vi "Main.vi"(11 "Module Admin":refnum<class "Delacor_lib_QMH_Module Admin.lvclass">) -> ()   [LabVIEW 2021, in "RT Interpreter Manager.lvlib"]
doc: "This template is based off of the Queued Message Handler design pattern and the Queued Message Handler project template that ships with LabVIEW.\n\nThe main difference is that the queue is private to this module and communication between modules is performed via Broadcast and Request events.\n\nRequest events are wrapped in public API methods and are handled in the Event Handling Loop (EHL) of this VI. Any module can register for Broadcast events sent by this module. The EHL generates messages based on user interface actions.\n\nThe Message Handling Loop (MHL) processes messages generated by the EHL, or by other messages. The messages are string values, so new messages can be added easily to the Message Cases case structure in the MHL. Each message cluster can also provide an optional value for Message Data, which is a variant that can be converted to whatever message-specific data is required.\n_____\nBased on DQMH Dev Tools: Project Template 7.1.2.1547."
uses:
  RT Interpreter Manager.lvlib
  <vilib>/Delacor/Delacor QMH/Libraries/Module Admin_class/Delacor_lib_QMH_Module Admin.lvclass
  Module Data--cluster.ctl
  Read Messages from Host HL--cluster.ctl
  Stop Argument--cluster.ctl
  <vilib>/Delacor/Delacor QMH/Libraries/Message Queue_class/Delacor_lib_QMH_Message Queue.lvclass/Delacor_lib_QMH_Message Queue.ctl
  <vilib>/Delacor/Delacor QMH/Libraries/Module Admin_class/Delacor_lib_QMH_Module Admin.lvclass/Delacor_lib_QMH_Module Admin.ctl
  New Host Connection Argument--cluster.ctl
  Send Message to Host Argument--cluster.ctl
  Libraries/UDP Comms/UDP Message--cluster.ctl
  Host/Host Interpreter/Host Initialization--cluster.ctl
  <vilib>/Utility/miscctls.llb/LVPointTypeDef.ctl
  0413ff4f-ab78-4adc-820c-bd9cd632877c.vi
  <vilib>/Delacor/Delacor QMH/Libraries/Message Queue_class/Delacor_lib_QMH_Enqueue Message (Single).vi
  <vilib>/Delacor/Delacor QMH/Libraries/Module Admin_class/Delacor_lib_QMH_Get External Launch.vi
  <vilib>/JDP Science/JSONtext/JSON text to Variant.vi
  <vilib>/JDP Science/JSONtext/LVClass Serializer/JSONtext LVClass Serializer.lvclass
  <vilib>/Delacor/Delacor QMH/Libraries/Message Queue_class/Delacor_lib_QMH_Message Queue.lvclass
  Libraries/Utilities/Utilities.lvlib
  RT Interpreter.lvlib
  Libraries/UDP Comms/UDP Comms.lvlib
  Libraries/Common RT/Common RT.lvlib
panel:
  out "error out":errorcluster
  out "Status":string
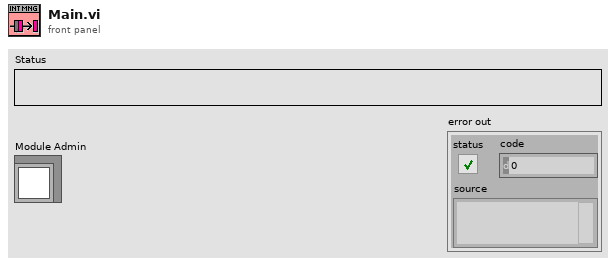
[diagram p1: front panel]
types:
  T1 = typedef "RT Interpreter Manager.lvlib/Request Events--cluster.ctl" = cluster{"Stop Module":refnum<user-event>, "Show Panel":refnum<user-event>, "Hide Panel":refnum<user-event>, "Get Module Execution Status":refnum<user-event>, "Show Diagram":refnum<user-event>, "Private.Get Config":refnum<user-event>, "Private.Open UDP":refnum<user-event>, "Private.Start Read Messages from Host HL":refnum<user-event>, "Private.New Host Connection":refnum<user-event>, "Private.Send Message to Host":refnum<user-event>, "Private.Delete Host Connection":refnum<user-event>}
  T2 = typedef "RT Interpreter Manager.lvlib/Read Messages from Host HL--cluster.ctl" = cluster{"Target UDP connection ID":refnum<k16>}
  T3 = typedef "RT Interpreter Manager.lvlib/Module Data--cluster.ctl" = cluster{"Status":string, "Target IP":string, "Target Listening Port":u16, "Polling Rate (ms)":i32, "UDP Connected?":bool, "Target UDP connection ID":refnum<k16>, "Host Connections IP:Port:Master/Slave":string[]}
  T4 = typedef "UDP Comms.lvlib/Host Initialization--cluster.ctl" = cluster{"Host IP":string, "Host Listening Port":u16, "MasterHost?":bool}
  T5 = enum32{"invalid lock state", "Not Locked", "Locked (No Password)", "Password-protected"}
  T6 = typedef "RT Interpreter Manager.lvlib/Stop Argument--cluster.ctl" = cluster{"Origin":string, "Exit via Stop Module Req?":bool, "Wait for Module to stop?":bool}
  T7 = typedef "RT Interpreter Manager.lvlib/New Host Connection Argument--cluster.ctl" = cluster{"Host Connection IP:Port:Master/Slave":string}
  T8 = typedef "RT Interpreter Manager.lvlib/Send Message to Host Argument--cluster.ctl" = cluster{"UDP Message":T9, "Remote IP":string, "Remote UDP Listening Port":u16}
  T9 = typedef "UDP Comms.lvlib/UDP Message--cluster.ctl" = cluster{"Command":string, "Data":variant}
  T10 = typedef "LVPointTypeDef.ctl" = cluster{"Horizontal":i16, "Vertical":i16}
  T11 = enum32{"Invalid", "Standard", "Closed", "Hidden", "Minimized", "Maximized"}
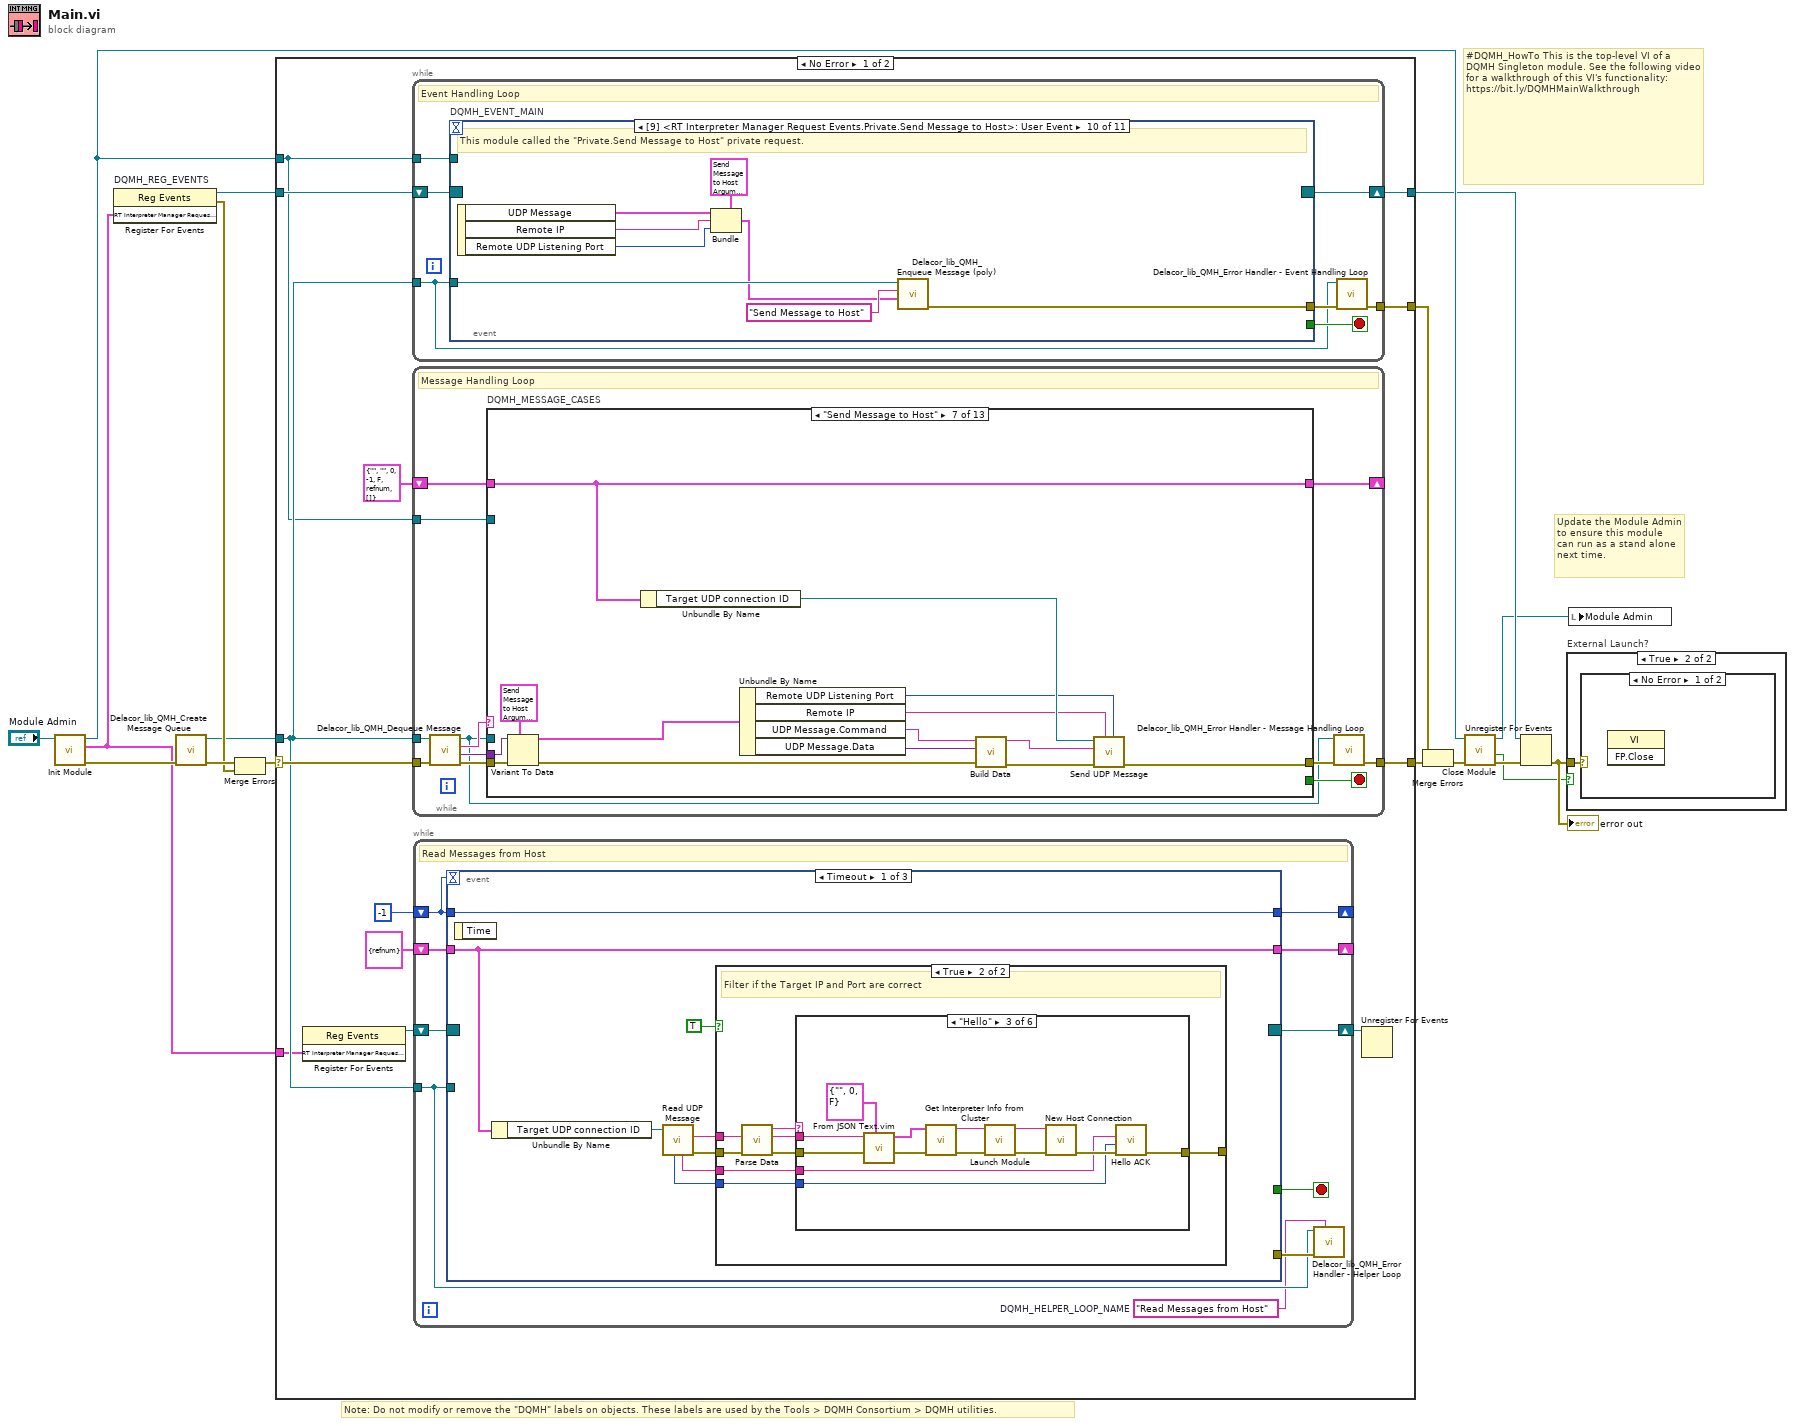
[diagram p0: block diagram]
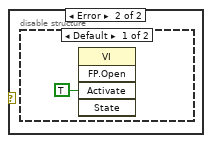
[diagram p3: hidden frame]
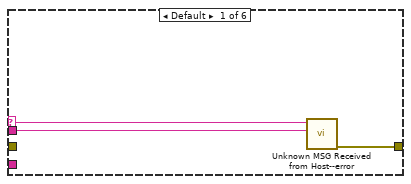
[diagram p6: hidden frame]
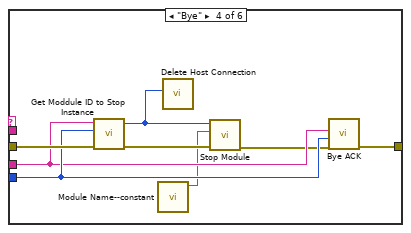
[diagram p8: hidden frame]
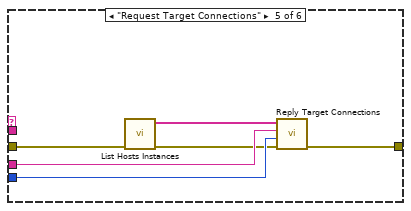
[diagram p9: hidden frame]
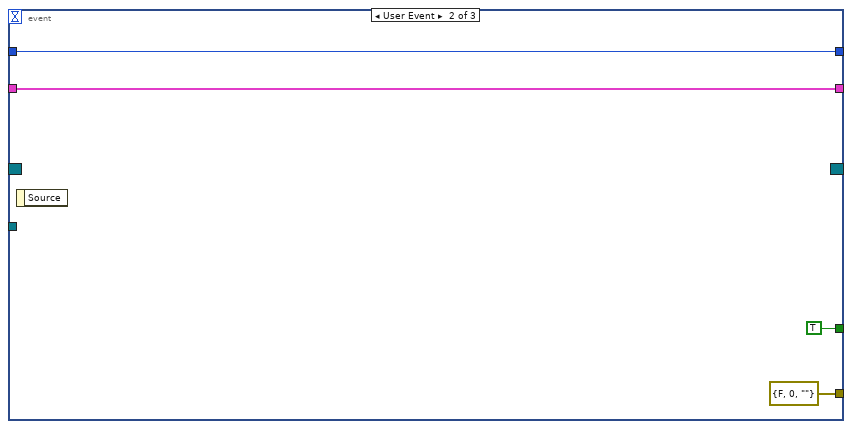
[diagram p11: hidden frame]
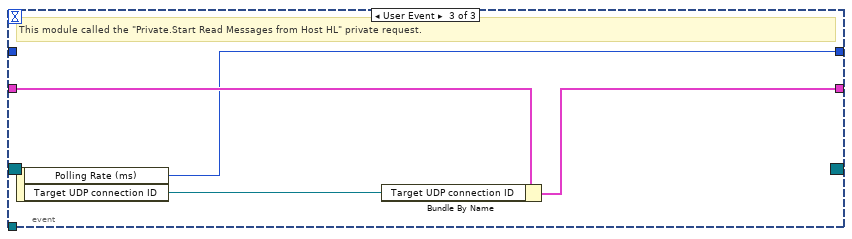
[diagram p12: hidden frame]
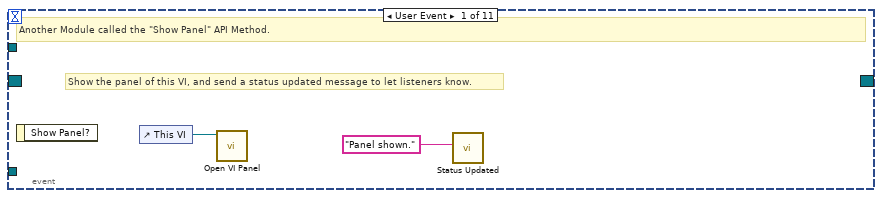
[diagram p13: hidden frame]
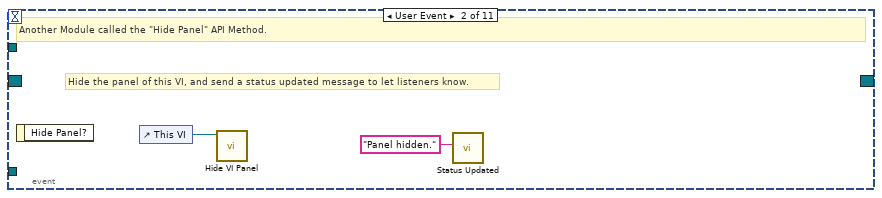
[diagram p14: hidden frame]
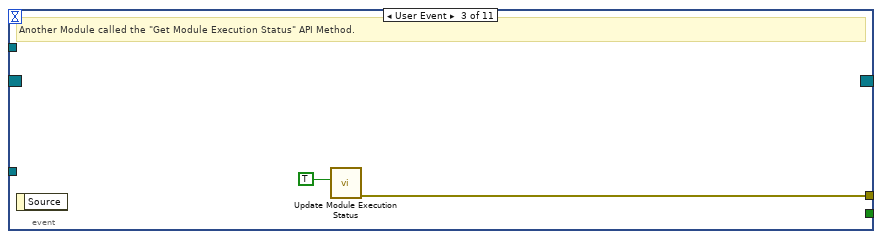
[diagram p15: hidden frame]
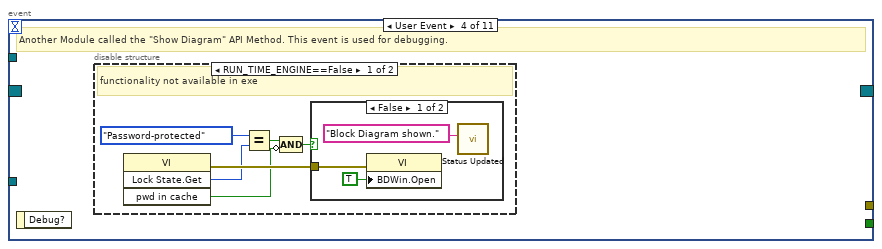
[diagram p16: hidden frame]
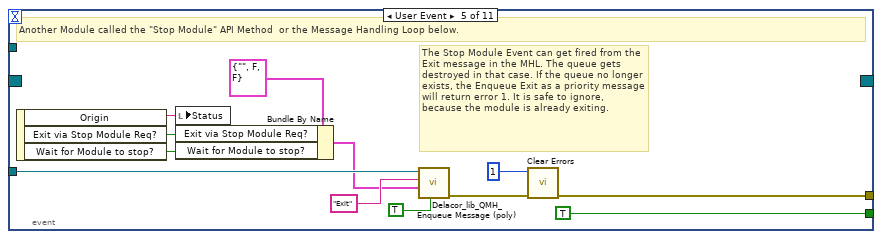
[diagram p19: hidden frame]
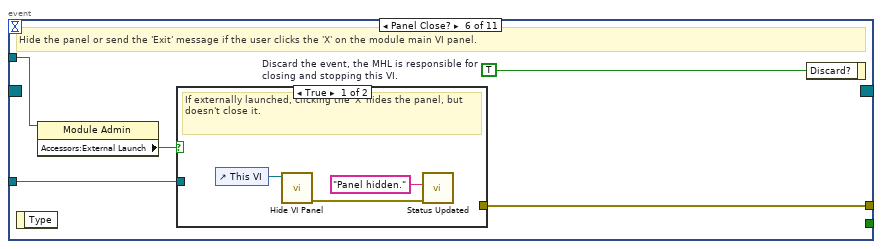
[diagram p20: hidden frame]
diagram:
  # "#DQMH_HowTo This is the top-level VI of a DQMH Singleton module. See the following video for a walkthrough of this VI's functionality: https://bit.ly/DQMHMainWalkthrough"
  # "Note: Do not modify or remove the \"DQMH\" labels on objects. These labels are used by the Tools > DQMH Consortium > DQMH utilities."
  # "Update the Module Admin to ensure this module can run as a stand alone next time."
  n1 = call "Init Module.vi"("Singleton Module Admin in"="Module Admin") -> ("error out"=w16:errorcluster, "RT Interpreter Manager Request Events"=w1:T1, "Singleton Module Admin out"=w8:refnum<class "Delacor_lib_QMH_Module Admin.lvclass">)  [unwired: 8 in]
  n2 = register-events "DQMH_REG_EVENTS"(w1) -> (reference out=w6:refnum<event-registration>, error out=w9:errorcluster)  [unwired: 2 in]
  n3 = call <vilib>:"Delacor_lib_QMH_Create Message Queue.vi"("error in"=w16) -> ("error out"=w11:errorcluster, "Message Queue"=w5:refnum<class "Delacor_lib_QMH_Message Queue.lvclass">)  [unwired: 9 in]
  n4 = Merge Errors(w11, w9) -> (w10:errorcluster)
  n5 = case shown="No Error" w10 {
    selector: w10 -> [w28 w316]
    tunnel: [w30 w315] -> w17
    tunnel: [w27 w314] -> w7
    tunnel: w6 -> [w25 w314]
    tunnel: w5 -> [w24 w309]
    tunnel: [w29 _] -> w14
    tunnel: w8 -> [w23 w310]
    tunnel: w1 -> [w22 _]
    frame No Error {
      n6 = register-events ("DQMH_HELPER_REGFOREVENTS")(w22) -> (reference out=w20:refnum<event-registration>)  [unwired: 2 in, 1 out]
      n7 = while {
        tunnel: w24 -> [w98]
        shift-right: [w101] -> w27
        shift-left: w25 -> [w102]
        tunnel: [w103] -> w29
        tunnel: w23 -> [w99]
        stop <- w100 stop-if-true
        # "Event Handling Loop"
        n8 = event "DQMH_EVENT_MAIN" shown="[9] <RT Interpreter Manager Request Events.Private.Send Message to Host>: User Event" {
          selector: w102 -> [_ _ _ _ _ _ _ _ _ _ _]
          dyn-events: [_ _ _ _ _ _ _ _ _ _ _] -> w101
          timeout: _ -> [_ _ _ _ _ _ _ _ _ _ _]
          tunnel: [_ _ _ _ TRUE ("Discard?") _ _ _ _ _ _] -> w100
          tunnel: w98 -> [_ _ _ _ w127 w134 w146 w149 w155 w163 w166]
          tunnel: [_ _ w110 _ w130 w136 w144 w147 w150 w158 w165] -> w104
          tunnel: w99 -> [_ _ _ _ _ w133 _ _ _ _ _]
          event User Event {
            # "Show the panel of this VI, and send a status updated message to let listeners know."
            # "Another Module called the \"Show Panel\" API Method."
            n9 = event-data() -> ()  [unwired: 1 in, 1 out]
            n10 = control-ref of="This VI"() -> (w106:refnum<vi>)
            n11 = call "Open VI Panel.vi"("VI"=w106) -> ()  [unwired: 10 in, 1 out]
            n12 = call "Status Updated.vi"("Status"="Panel shown." ("format string")) -> ()  [unwired: 10 in, 1 out]
          }
          event User Event {
            # "Hide the panel of this VI, and send a status updated message to let listeners know."
            # "Another Module called the \"Hide Panel\" API Method."
            n13 = event-data() -> ()  [unwired: 1 in, 1 out]
            n14 = control-ref of="This VI"() -> (w108:refnum<vi>)
            n15 = call "Hide VI Panel.vi"("VI"=w108) -> ()  [unwired: 10 in, 1 out]
            n16 = call "Status Updated.vi"("Status"="Panel hidden." ("format string")) -> ()  [unwired: 10 in, 1 out]
          }
          event User Event {
            # "Another Module called the \"Get Module Execution Status\" API Method."
            n17 = event-data() -> ()  [unwired: 1 in, 1 out]
            n18 = call "Update Module Execution Status.vi"("Running?"=TRUE) -> ("error out"=w110:errorcluster)  [unwired: 10 in]
          }
          event User Event {
            # "Another Module called the \"Show Diagram\" API Method. This event is used for debugging."
            n19 = event-data() -> ()  [unwired: 1 in, 1 out]
            n20 = disable-structure shown="RUN_TIME_ENGINE==False" {
              frame condition #0 (active) {
                # "functionality not available in exe"
                n21 = invoke on="Invoke Node" class="VI" method="Lock State.Get"() -> (error out=w116:errorcluster, "Get Lock State"=w115:T5, "pwd in cache"=w112:bool)  [unwired: 4 in, 1 out]
                n22 = Equal?(x=T5."Password-protected", y=w115) -> (x = y?=w113:bool)
                n23 = Compound Arithmetic op=AND(w113, invert w112) -> (w111:bool)
                n24 = case shown="False" w111 {
                  tunnel: w116 -> [w119 _]
                  frame False {
                    n25 = property on="Property Node" class="VI"(error in=w119, "BDWin.Open"=TRUE ("Block Diagram Window:Open")) -> ()  [unwired: 1 in, 2 out]
                    n26 = call "Status Updated.vi"("Status"="Block Diagram shown." ("format string")) -> ()  [unwired: 10 in, 1 out]
                  }
                  frame True {
                    # "Password-protected VI, and the password is not in the cache. Do not show the diagram."
                  }
                }
              }
              frame condition #1 {
              }
            }
          }
          event User Event {
            # "The Stop Module Event can get fired from the Exit message in the MHL. The queue gets destroyed in that case. If the queue no longer exists, the Enqueue Exit as a priority message will return error 1. It is safe to ignore, because the module is already exiting."
            # "Another Module called the \"Stop Module\" API Method  or the Message Handling Loop below."
            n27 = event-data() -> ("Origin"=w126:string, "Exit via Stop Module Req?"=w122:bool, "Wait for Module to stop?"=w121:bool)  [unwired: 1 in]
            n28 = local write "Status"(w126) -> ()
            n29 = Bundle By Name(cluster=T6 {"Origin"="", "Exit via Stop Module Req?"=FALSE, "Wait for Module to stop?"=FALSE} ("Stop Argument"), "Exit via Stop Module Req?"=w122, "Wait for Module to stop?"=w121) -> (w120:T6)
            n30 = call-poly <vilib>:"Delacor_lib_QMH_Enqueue Message (poly).vi"("Priority Message? (F)"=TRUE, "Message Data"=w120, "Message"="Exit", "Message Queue in"=w127) -> ("error out"=w131:errorcluster)  [unwired: 6 in, 1 out]
            n31 = call <vilib>:"Clear Errors.vi"("error in (no error)"=w131, "specific error code to clear (0: all)"=1) -> ("error out"=w130:errorcluster)  [unwired: 4 in, 1 out]
          }
          event Panel Close? {
            w135 = TRUE  # Discard the event, the MHL is responsible for closing and stopping this VI.
            # "Hide the panel or send the 'Exit' message if the user clicks the 'X' on the module main VI panel."
            n32 = event-data() -> ()  [unwired: 1 in, 1 out]
            n33 = property on="Property Node" class="Module Admin"(reference=w133) -> ("Accessors:External Launch"=w132:bool)  [unwired: 1 in, 2 out]
            n34 = case shown="True" w132 {
              tunnel: w134 -> [_ w142]
              tunnel: [_ w143] -> w136
              frame True {
                # "If externally launched, clicking the 'X' hides the panel, but doesn't close it."
                n35 = control-ref of="This VI"() -> (w139:refnum<vi>)
                n36 = call "Hide VI Panel.vi"("VI"=w139) -> ("error out"=w137:errorcluster)  [unwired: 10 in]
                n37 = call "Status Updated.vi"("error in"=w137, "Status"="Panel hidden." ("format string")) -> ()  [unwired: 9 in, 1 out]
              }
              frame False {
                # "If run as a stand-alone VI, clicking the panel 'X' stops the VI."
                n38 = call-poly <vilib>:"Delacor_lib_QMH_Enqueue Message (poly).vi"("Priority Message? (F)"=TRUE, "Message"="Exit", "Message Queue in"=w142) -> ("error out"=w143:errorcluster)  [unwired: 7 in, 1 out]
              }
            }
            n39 = event-data ("Event Filter Node")("Discard?"=w135) -> ()  [unwired: 1 in, 1 out]
          }
          event User Event {
            # "This module called the \"Private.Get Config\" private request."
            n40 = event-data() -> ()  [unwired: 1 in, 1 out]
            n41 = call-poly <vilib>:"Delacor_lib_QMH_Enqueue Message (poly).vi"("Message"="Get Config", "Message Queue in"=w146) -> ("error out"=w144:errorcluster)  [unwired: 8 in, 1 out]
          }
          event User Event {
            # "This module called the \"Private.Open UDP\" private request."
            n42 = event-data() -> ()  [unwired: 1 in, 1 out]
            n43 = call-poly <vilib>:"Delacor_lib_QMH_Enqueue Message (poly).vi"("Message"="Open UDP", "Message Queue in"=w149) -> ("error out"=w147:errorcluster)  [unwired: 8 in, 1 out]
          }
          event User Event {
            # "This module called the \"Private.New Host Connection\" private request."
            n44 = event-data() -> ("Host Connection IP:Port:Master/Slave"=w151:string)  [unwired: 1 in]
            n45 = Bundle(cluster=T7 {"Host Connection IP:Port:Master/Slave"=""} ("New Host Connection Argument"), "Host Connection IP:Port:Master/Slave"=w151) -> (w152:T7)
            n46 = call-poly <vilib>:"Delacor_lib_QMH_Enqueue Message (poly).vi"("Message Data"=w152, "Message"="New Host Connection", "Message Queue in"=w155) -> ("error out"=w150:errorcluster)  [unwired: 7 in, 1 out]
          }
          event User Event {
            # "This module called the \"Private.Send Message to Host\" private request."
            n47 = event-data() -> ("UDP Message"=w159:T9, "Remote IP"=w157:string, "Remote UDP Listening Port"=w156:u16)  [unwired: 1 in]
            n48 = Bundle(cluster=T8 {"UDP Message"={"Command"="", "Data"=variant}, "Remote IP"="", "Remote UDP Listening Port"=0} ("Send Message to Host Argument"), "UDP Message"=w159, "Remote IP"=w157, "Remote UDP Listening Port"=w156) -> (w160:T8)
            n49 = call-poly <vilib>:"Delacor_lib_QMH_Enqueue Message (poly).vi"("Message Data"=w160, "Message"="Send Message to Host", "Message Queue in"=w163) -> ("error out"=w158:errorcluster)  [unwired: 7 in, 1 out]
          }
          event User Event {
            n50 = event-data() -> ("index of host connection"=w164:i32)  [unwired: 1 in]
            n51 = call-poly <vilib>:"Delacor_lib_QMH_Enqueue Message (poly).vi"("Message Data"=w164, "Message"="Delete host connection", "Message Queue in"=w166) -> ("error out"=w165:errorcluster)  [unwired: 7 in, 1 out]
          }
        }
        n52 = call-dynamic "Delacor_lib_QMH_Error Handler - Event Handling Loop.vi"("error in"=w104, "Message Queue in"=w98) -> ("dup error in"=w103:errorcluster)  [unwired: 8 in, 1 out]
      }
      n53 = while {
        tunnel: w24 -> [w168]
        shift-right: [w176] -> _
        shift-left: T3 {"Status"="", "Target IP"="", "Target Listening Port"=0, "Polling Rate (ms)"=-1, "UDP Connected?"=FALSE, "Target UDP connection ID"=refnum, "Host Connections IP:Port:Master/Slave"=[]} ("Data Cluster") -> [w177]
        tunnel: w28 -> [w179]
        tunnel: [w171] -> w30
        tunnel: w23 -> [w172]
        stop <- w175 stop-if-true
        # "Message Handling Loop"
        n54 = call-dynamic "Delacor_lib_QMH_Dequeue Message.vi"("error in"=w179, "Message Queue in"=w168) -> ("error out"=w178:errorcluster, "Message Data"=w173:variant, "Message"=w174:string, "Message Queue out"=w169:refnum<class "Delacor_lib_QMH_Message Queue.lvclass">)  [unwired: 6 in]
        n55 = case "DQMH_MESSAGE_CASES" shown="\"Send Message to Host\"" w174 {
          selector: w174 -> [_ _ _ _ _ _ _ _ _ _ _ _ w304]
          tunnel: w169 -> [_ _ _ _ _ _ _ _ _ _ w270 w292 _]
          tunnel: w178 -> [w198 w202 w204 w215 w228 w238 w252 w255 w257 w266 w277 w298 w307]
          tunnel: [w197 w202 w203 w214 w227 w237 w244 w254 w257 w265 w273 w293 w308] -> w170
          tunnel: w177 -> [w188 w201 w209 w213 w223 w234 w242 w253 w256 w263 w272 w291 w305]
          tunnel: [w187 w201 w208 w212 w222 w233 w242 w253 w256 w263 w272 w291 w305] -> w176
          tunnel: [_ _ _ _ _ _ _ _ _ _ _ w290 _] -> w175
          tunnel: w173 -> [_ _ _ _ w226 w236 w251 _ _ _ w271 w289 _]
          tunnel: w172 -> [w189 _ _ _ _ _ _ _ _ _ w269 w284 _]
          frame "Initialize" {
            w183 = "Initial Message" ("Initial Message")
            # "Initialize - Any operation that needs to be done before the module can receive messages. Synchronize Caller Events.vi will inform Start Module.vi that the module has launched and is ready to receive messages. Module Did Init.vi will broadcast that the module initialized."
            n56 = call "Synchronize Caller Events.vi"("error in"=w198, "Singleton Module Admin in"=w189) -> ("error out"=w180:errorcluster, "Singleton Module Admin out"=w184:refnum<class "Delacor_lib_QMH_Module Admin.lvclass">)  [unwired: 8 in]
            n57 = property on="Property Node" class="Module Admin"(reference=w184) -> ("Accessors:External Launch"=w193:bool)  [unwired: 1 in, 2 out]
            n58 = Select(t=T11."Hidden" ("State"), s=w193, f=T11."Standard" ("State")) -> (s? t:f=w190:T11)
            n59 = call "Module Name--constant.vi"() -> ("Module Name"=w196:string)  [unwired: 11 in]
            n60 = property on="Property Node" class="VI"("Front Panel.Title"=w196) -> (reference out=w195:refnum<vi>, error out=w200:errorcluster)  [unwired: 2 in]
            n61 = invoke on="Invoke Node" class="VI" method="FP.Open"(reference=w195, error in=w200, "State"=w190) -> (reference out=w194:refnum<vi>, error out=w199:errorcluster)  [unwired: 2 in, 3 out]
            n62 = Bundle By Name(cluster=w188, "Status"=w183) -> (w187:T3)
            n63 = invoke on="Invoke Node" class="VI" method="FP.Center"(reference=w194, error in=w199) -> ()  [unwired: 1 in, 3 out]
            n64 = property on="Pane" class="Pane"("Origin"=T10 {"Horizontal"=0, "Vertical"=0}) -> ()  [unwired: 2 in, 2 out]
            n65 = call "Get Config.vi"("error in"=w180) -> ("error out"=w181:errorcluster)  [unwired: 10 in]
            n66 = call "Module Name--constant.vi"() -> ("Module Name"=w185:string)  [unwired: 11 in]
            n67 = call "Module Did Init.vi"("error in"=w181, "Initialized?"=TRUE, "Origin"=w185) -> ("error out"=w197:errorcluster)  [unwired: 8 in]
            "Status" <- w183
          }
          frame "---Module Specific---" {
            # "Separator -- The following cases handle messages specific to this Module."
          }
          frame "Get Config" {
            n68 = call "Get Local IP.vi"() -> ("Local IP"=w207:string)  [unwired: 4 in]
            n69 = Bundle By Name(cluster=w209, "Target IP"=w207, "Target Listening Port"=u16 61670 ("Port RT"), "Polling Rate (ms)"=50) -> (w208:T3)
            n70 = call "Open UDP.vi"("error in"=w204) -> ("error out"=w203:errorcluster)  [unwired: 10 in]
          }
          frame "Open UDP" {
            n71 = Unbundle By Name(w213) -> ("Polling Rate (ms)"=w211:i32, "Target IP"=w217:string, "Target Listening Port"=w218:u16)
            n72 = String To IP(1:w217) -> (0:w216:u32)
            n73 = UDP Open(7:w216, 8:w215, 11:w218) -> (port=w210:refnum<k16>, 0:w214:errorcluster)  [unwired: 2 in, 1 out]
            n74 = Bundle By Name(cluster=w213, "Target UDP connection ID"=w210) -> (w212:T3)
            n75 = call "Start Read Messages from Host HL.vi"("Target UDP connection ID"=w210, "Polling Rate (ms)"=w211) -> ()  [unwired: 9 in, 1 out]
          }
          frame "New Host Connection" {
            n76 = Variant To Data(error in=w228, type=T7 {"Host Connection IP:Port:Master/Slave"=""} ("New Host Connection Argument"), Variant=w226) -> (data=w224:T7, error out=w227:errorcluster)
            n77 = Unbundle By Name(w224) -> ("Host Connection IP:Port:Master/Slave"=w220:string)
            n78 = Unbundle By Name(w223) -> ("Host Connections IP:Port:Master/Slave"=w221:string[])
            n79 = Build Array (concatenate)(w221, w220) -> (w219:string[])
            n80 = Bundle By Name(cluster=w223, "Host Connections IP:Port:Master/Slave"=w219) -> (w222:T3)
          }
          frame "Delete host connection" {
            n81 = Variant To Data(error in=w238, type=0 ("index of host connection"), Variant=w236) -> (data=w231:i32, error out=w237:errorcluster)
            n82 = Unbundle By Name(w234) -> ("Host Connections IP:Port:Master/Slave"=w232:string[])
            n83 = Delete From Array(array=w232, length=0, index=w231) -> (array with subset deleted=w229:string[])  [unwired: 1 out]
            n84 = Bundle By Name(cluster=w234, "Host Connections IP:Port:Master/Slave"=w229) -> (w233:T3)
          }
          frame "Send Message to Host" {
            n85 = Variant To Data(error in=w252, type=T8 {"UDP Message"={"Command"="", "Data"=variant}, "Remote IP"="", "Remote UDP Listening Port"=0} ("Send Message to Host Argument"), Variant=w251) -> (data=w243:T8, error out=w245:errorcluster)
            n86 = Unbundle By Name(w242) -> ("Target UDP connection ID"=w241:refnum<k16>)
            n87 = Unbundle By Name(w243) -> ("Remote UDP Listening Port"=w240:u16, "Remote IP"=w239:string, "UDP Message.Command"=w248:string, "UDP Message.Data"=w247:variant)
            n88 = call "Build Data.vi"("error in (no error)"=w245, "Data"=w247, "Command"=w248) -> ("error out"=w249:errorcluster, "UDP MSG To be Sent"=w246:string)  [unwired: 7 in]
            n89 = call "Send UDP Message.vi"("Remote UDP Listening Port"=w240, "Remote IP"=w239, "error in"=w249, "UDP Data to be sent"=w246, "Local UDP connection ref"=w241) -> ("error out"=w244:errorcluster)  [unwired: 5 in, 1 out]
          }
          frame "---Copy This Frame---" {
            # "Duplicate this frame when creating new messages.  Change this comment in the duplicated frame to describe this message."
            n90 = Merge Errors(w255) -> (w254:errorcluster)
          }
          frame "---Exit and Error Handling---" {
            # "Separator - The following cases handle errors and exit messages."
          }
          frame "Simulate MHL Error" {
            # "#DQMH_HowTo The 'Simulate MHL Error' button  illustrates how the MHL handles errors. This event is instructional in nature and can be removed."
            # "Simulate an error occurring at the MHL"
            n91 = call "Module Name--constant.vi"() -> ("Module Name"=w259:string)  [unwired: 11 in]
            n92 = Format Into String(format string="Simulated error originating at Message Handling Loop in %s", w259) -> (resulting string=w260:string)  [unwired: 2 in, 1 out]
            n93 = call <vilib>:"Error Cluster From Error Code.vi"("show call chain? (False)"=TRUE, "error message (\"\")"=w260, "error code (0)"=5001) -> ("error out"=w264:errorcluster)  [unwired: 6 in]
            n94 = Merge Errors(w266, w264) -> (w265:errorcluster)
          }
          frame "Error" {
            # "#DQMH_CodeRecommended - If the module is running in standalone mode (External Launch = FALSE), this code will pop up an error dialog and call the 'Exit' message if an error occurs. Add more fine-grained error management here."
            # "Error - Check the error message data and respond accordingly. This message is sent by the \"Error Handler\" VIs at the end of each loop in this application."
            n95 = property on="Property Node" class="Module Admin"(reference=w269) -> ("Accessors:External Launch"=w268:bool)  [unwired: 1 in, 2 out]
            n96 = Variant To Data(error in=w277, type=errorcluster {"status"=FALSE, "code"=0, "source"=""} ("error constant"), Variant=w271) -> (data=w267:errorcluster, error out=w275:errorcluster)
            n97 = local write "error out"(w267) -> ()
            n98 = call "Error Reported.vi"("Error"=w267) -> ()  [unwired: 10 in, 1 out]
            n99 = case shown="False" w268 {
              tunnel: [w282 _] -> w274
              tunnel: w270 -> [w280 _]
              tunnel: w267 -> [w281 _]
              frame False {
                n100 = disable-structure shown="Default" {
                  disable-tunnel: w281 -> [w283 _]
                  frame condition #0 (active) {
                    # "If the module is running standalone, then pop up an error dialog and call the \"Exit\" message."
                    n101 = call <vilib>:"Simple Error Handler.vi"("error in (no error)"=w283) -> ()  [unwired: 4 in, 5 out]
                  }
                  frame condition #1 {
                    # "To prevent the Simple Error Handler VI from being loaded (e.g. when deploying to a Real-Time target), add the Conditional Disable Symbol \"DQMH_Disable_SEH\" to your project and set it to TRUE."
                  }
                }
                n102 = call-poly <vilib>:"Delacor_lib_QMH_Enqueue Message (poly).vi"("Priority Message? (F)"=TRUE, "Message"="Exit", "Message Queue in"=w280) -> ("error out"=w282:errorcluster)  [unwired: 7 in, 1 out]
              }
              frame True {
                # "If the module was launched externally, calling the Error Reported broadcast VI is the only action performed by the \"Error\" message. The module's caller can then process the error appropriately."
              }
            }
            n103 = Merge Errors(w275, w274) -> (w273:errorcluster)
          }
          frame "Exit" {
            w288 = 91  # 91: not all Exit messages will have an argument
            w290 = TRUE  # Stop the VI
            # "Release the message queue reference"
            # "#DQMH_CodeNeeded - Add any required cleanup code here."
            # "Exit - Exit the application."
            n104 = Variant To Data(error in=w298, type=T6 {"Origin"="", "Exit via Stop Module Req?"=FALSE, "Wait for Module to stop?"=FALSE} ("Stop Argument"), Variant=w289) -> (data=w286:T6, error out=w295:errorcluster)
            n105 = call <vilib>:"Clear Errors.vi"("error in (no error)"=w295, "specific error code to clear (0: all)"=w288) -> ("error out"=w297:errorcluster)  [unwired: 4 in, 1 out]
            n106 = control-ref of="This VI"() -> (w285:refnum<vi>)
            n107 = call-dynamic "Delacor_lib_QMH_Release Message Queue.vi"("error in"=w297, "Message Queue"=w292) -> ("error out"=w296:errorcluster)  [unwired: 9 in]
            n108 = call "Handle Exit.vi"("Stop Argument"=w286, "Admin in"=w284, "VI reference"=w285) -> ("error out"=w294:errorcluster)  [unwired: 7 in, 1 out]
            n109 = Merge Errors(w296, w294) -> (w293:errorcluster)
            n110 = call "Error Reported.vi"("Error"=w293) -> ()  [unwired: 10 in, 1 out]
          }
          frame Default {
            # "'Default' case only runs if there is a message that isn't defined in any of the other cases.  Output a programming error."
            n111 = call "Module Name--constant.vi"() -> ("Module Name"=w303:string)  [unwired: 11 in]
            n112 = Format Into String(format string="The invalid message string \"%s\" was received in the Message Handling Loop for module \"%s\".", w304, w303) -> (resulting string=w299:string)  [unwired: 2 in, 1 out]
            n113 = call <vilib>:"Error Cluster From Error Code.vi"("show call chain? (False)"=TRUE, "error message (\"\")"=w299, "error code (0)"=1) -> ("error out"=w306:errorcluster)  [unwired: 6 in]
            n114 = Merge Errors(w307, w306) -> (w308:errorcluster)
          }
        }
        n115 = call-dynamic "Delacor_lib_QMH_Error Handler - Message Handling Loop.vi"("error in"=w170, "Message Queue in"=w169) -> ("dup error in"=w171:errorcluster)  [unwired: 8 in, 1 out]
      }
      n116 = while "DQMH_HELPER_LOOP" {
        shift-right: [w40] -> _
        shift-left: -1 -> [w39]
        shift-right: [w37] -> w21
        shift-left: w20 -> [w38]
        tunnel: w24 -> [w34]
        shift-right: [w31] -> _
        shift-left: T2 {"Target UDP connection ID"=refnum} ("Read Messages from Host HL--cluster") -> [w32]
        stop <- w36 stop-if-true
        w33 = "Read Messages from Host"  # DQMH_HELPER_LOOP_NAME
        # "Read Messages from Host"
        n117 = event "DQMH_HELPER_EVENT_STRUCTURE" shown="[0] Timeout" {
          selector: w38 -> [_ _ _]
          dyn-events: [_ _ _] -> w37
          timeout: w39 -> [_ _ _]
          tunnel: w39 -> [w48 w93 _]
          tunnel: [w48 w93 w94] -> w40
          tunnel: [_ TRUE _] -> w36
          tunnel: [_ errorcluster {"status"=FALSE, "code"=0, "source"=""} ("error constant") _] -> w35
          tunnel: w34 -> [_ _ _]
          tunnel: w32 -> [w47 w90 w97]
          tunnel: [w47 w90 w96] -> w31
          event Timeout {
            n118 = event-data() -> ()  [unwired: 1 in, 1 out]
            n119 = Unbundle By Name(w47) -> ("Target UDP connection ID"=w43:refnum<k16>)
            n120 = call "Read UDP Message.vi"("Local UDP connection ref"=w43) -> ("error out"=w46:errorcluster, "data out"=w45:string, "Remote IP"=w42:string, "Remote Port"=w41:u16)  [unwired: 6 in, 1 out]
            n121 = case shown="True" TRUE {
              tunnel: w46 -> [w49 w57]
              tunnel: w45 -> [_ w56]
              tunnel: [w49 w52] -> _
              tunnel: w42 -> [_ w51]
              tunnel: w41 -> [_ w50]
              frame False {
              }
              frame True {
                # "Filter if the Target IP and Port are correct"
                n122 = call "Parse Data.vi"("error in (no error)"=w57, "Received UDP Data"=w56) -> ("error out"=w54:errorcluster, "Data"=w53:string, "Command"=w55:string)  [unwired: 7 in]
                n123 = case shown="\"Hello\"" w55 {
                  selector: w55 -> [w59 _ _ _ _ _]
                  tunnel: w54 -> [_ w61 w74 w81 w85 w89]
                  tunnel: w53 -> [w58 _ w72 _ _ _]
                  tunnel: [w60 w61 w64 w82 w88 w89] -> w52
                  tunnel: w51 -> [_ _ w62 w79 w87 _]
                  tunnel: w50 -> [_ _ w63 w80 w86 _]
                  frame Default {
                    n124 = call "Unknown MSG Received from Host--error.vi"("Data"=w58, "Command"=w59) -> ("error out"=w60:errorcluster)  [unwired: 9 in]
                  }
                  frame "--- MSGs from Host ---" {
                  }
                  frame "Hello" {
                    n125 = call "From JSON Text.vim"("Data Type and Default Value"=T4 {"Host IP"="", "Host Listening Port"=0, "MasterHost?"=FALSE} ("Host Initialization--cluster"), "error in (no error)"=w74, "JSON"=w72) -> ("error out"=w71:errorcluster, "Data out"=w68:T4)  [unwired: 7 in]
                    n126 = call "Get Interpreter Info from Cluster.vi"("error in"=w71, "Host Initialization--cluster"=w68) -> ("error out"=w69:errorcluster, "IP:Port:Master/Slave"=w70:string)  [unwired: 8 in]
                    n127 = call "Launch Module.vi"("error in"=w69, "IP:Port:Master/Slave"=w70) -> ("error out"=w67:errorcluster, "IP:Port:Master/Slave out"=w66:string)  [unwired: 8 in]
                    n128 = call "New Host Connection.vi"("error in"=w67, "Host Connection IP:Port:Master/Slave"=w66) -> ("error out"=w65:errorcluster)  [unwired: 9 in]
                    n129 = call "Hello ACK.vi"("error in"=w65, "Remote UDP Listening Port"=w63, "Remote IP"=w62) -> ("error out"=w64:errorcluster)  [unwired: 8 in]
                  }
                  frame "Bye" {
                    n130 = call "Get Moddule ID to Stop Instance.vi"("error in"=w81, "Remote Port"=w80, "Remote IP"=w79) -> ("error out"=w78:errorcluster, "Module ID to be deleted"=w75:i32)  [unwired: 6 in, 1 out]
                    n131 = call "Module Name--constant.vi"() -> ("Module Name"=w76:string)  [unwired: 11 in]
                    n132 = call "Delete Host Connection.vi"("index of host connection"=w75) -> ()  [unwired: 10 in, 1 out]
                    n133 = call "Stop Module.vi"("error in"=w78, "Origin"=w76, "Module ID"=w75) -> ("error out"=w77:errorcluster)  [unwired: 8 in]
                    n134 = call "Bye ACK.vi"("error in"=w77, "Remote UDP Listening Port"=w80, "Remote IP"=w79) -> ("error out"=w82:errorcluster)  [unwired: 8 in]
                  }
                  frame "Request Target Connections" {
                    n135 = call "List Hosts Instances.vi"("error in"=w85) -> ("error out"=w83:errorcluster, "List of IP:Port:Master/Slave"=w84:string[])  [unwired: 9 in]
                    n136 = call "Reply Target Connections.vi"("error in"=w83, "Remote UDP Listening Port"=w86, "Remote IP"=w87, "List of IP:Port:Master/Slave"=w84) -> ("error out"=w88:errorcluster)  [unwired: 7 in]
                  }
                  frame "--- ACK MSGs ---" {
                  }
                }
              }
            }
          }
          event User Event {
            n137 = event-data() -> ()  [unwired: 1 in, 1 out]
          }
          event User Event {
            # "This module called the \"Private.Start Read Messages from Host HL\" private request."
            n138 = event-data() -> ("Polling Rate (ms)"=w94:i32, "Target UDP connection ID"=w95:refnum<k16>)  [unwired: 1 in]
            n139 = Bundle By Name(cluster=w97, "Target UDP connection ID"=w95) -> (w96:T2)
          }
        }
        n140 = call-dynamic "Delacor_lib_QMH_Error Handler - Helper Loop.vi"("Error Debug"=w33, "error in"=w35, "Message Queue in"=w34) -> ()  [unwired: 7 in, 2 out]
      }
      n141 = Unregister For Events(event registration refnum=w21) -> ()  [unwired: 1 in, 1 out]
    }
    frame Error {
      # "Synchronize Caller Events.vi will inform Start Module.vi that the module has launched and will let the code calling Start Module.vi register for broadcasts and would permit the caller receive the broadcast that an error occurred at launch time."
      n142 = call-dynamic "Delacor_lib_QMH_Release Message Queue.vi"("error in"=w316, "Message Queue"=w309) -> ("error out"=w315:errorcluster)  [unwired: 9 in]
      n143 = call "Synchronize Caller Events.vi"("Singleton Module Admin in"=w310) -> ("error out"=w317:errorcluster)  [unwired: 9 in, 1 out]
      n144 = call "Module Name--constant.vi"() -> ("Module Name"=w313:string)  [unwired: 11 in]
      n145 = Format Into String(format string="An error occurred during initialization. %s is no longer running.", w313) -> (resulting string=w311:string)  [unwired: 2 in, 1 out]
      n146 = Merge Errors(w315, w317) -> (w318:errorcluster)
      n147 = call "Error Reported.vi"("Additional Information"=w311, "Error"=w318) -> ()  [unwired: 9 in, 1 out]
    }
  }
  n148 = Merge Errors(w14, w17) -> (w13:errorcluster)
  n149 = call "Close Module.vi"("error in"=w13, "Module Admin in"=w8) -> ("error out"=w15:errorcluster, "External Launch"=w2:bool, "Module Admin out"=w3:refnum<class "Delacor_lib_QMH_Module Admin.lvclass">)  [unwired: 7 in]
  n150 = Unregister For Events(event registration refnum=w7, error in=w15) -> (error out=w12:errorcluster)
  "error out" <- w12
  n151 = case "External Launch?" shown="True" w2 {
    tunnel: w12 -> [_ w319]
    frame False {
    }
    frame True {
      n152 = case shown="No Error" w319 {
        frame No Error {
          n153 = invoke on="Invoke Node" class="VI" method="FP.Close"() -> ()  [unwired: 3 in, 3 out]
        }
        frame Error {
          n154 = disable-structure shown="Default" {
            frame condition #0 (active) {
              n155 = invoke class="VI" method="FP.Open"("Activate"=TRUE ("Activate?")) -> ()  [unwired: 4 in, 5 out]
            }
            frame condition #1 {
              # "Don't show panel on error if running inside a built EXE."
            }
          }
        }
      }
    }
  }
  n156 = local write "Module Admin"(w3) -> ()
